vi "Pupil&CR_Detecter.vi"(8 "Image Name":string="ellipse2", 9 "Pupil Threshold":u8=10, 10 "HighLight Spot Threshold":u8=220, 11 "image input":T2) -> (0 "valid fit":T3, 1 "Image Dst Out":T2, 2 "pupil Circles Data":cluster{"Pos. X":sgl, "Pos. Y":sgl}, 3 "CR Circles Data":cluster{"Pos. X":sgl, "Pos. Y":sgl}, 4 "Image Out":T2, 5 "Axis":T1)   [LabVIEW 2011]
uses:
  <vilib>/vision/Image Controls.llb/IMAQ Image.ctl
  <vilib>/vision/NI_Vision_Development_Module.lvlib
panel:
  out "Point 1":cluster{"X":sgl, "Y":sgl}
  out "Point 2":cluster{"X":sgl, "Y":sgl}
  out "CR Valid Fit 2":bool
  out "Pupil Valid Fit":bool
  in  "Size & Tolerance":T4={"X Size"=4, "Y Size"=4, "% Tolerance"=0}
  out "pupil Nb Circles":i32
  in  "CR Max Radius":sgl=10.0 format="%.2f"
  in  "CR Min Radius":sgl=2.0 format="%.2f"
  out "CR Nb Circles":i32
  in  "CR Operator":T5(ring)
  in  "edge Operator":T5(ring)
  in  "edge Range":cluster{"Minimum":sgl, "Maximum":sgl}={"Minimum"=254.0, "Maximum"=255.0} {"Maximum" format="%.2f"; "Minimum" format="%.2f"}
  in  "pupil find edge Method":T6(ring)
  in  "pupil find edge Threshold Value":sgl
  in  "pupil OI Operator":T5(ring)=enum."Square"
  in  "pupil Max Radius":sgl=50.0
  in  "pupil Min Radius":sgl=10.0
  # "step2"
  # "step1"
  # "step1"
  # "step2"
  # "step3"
  # "step4"
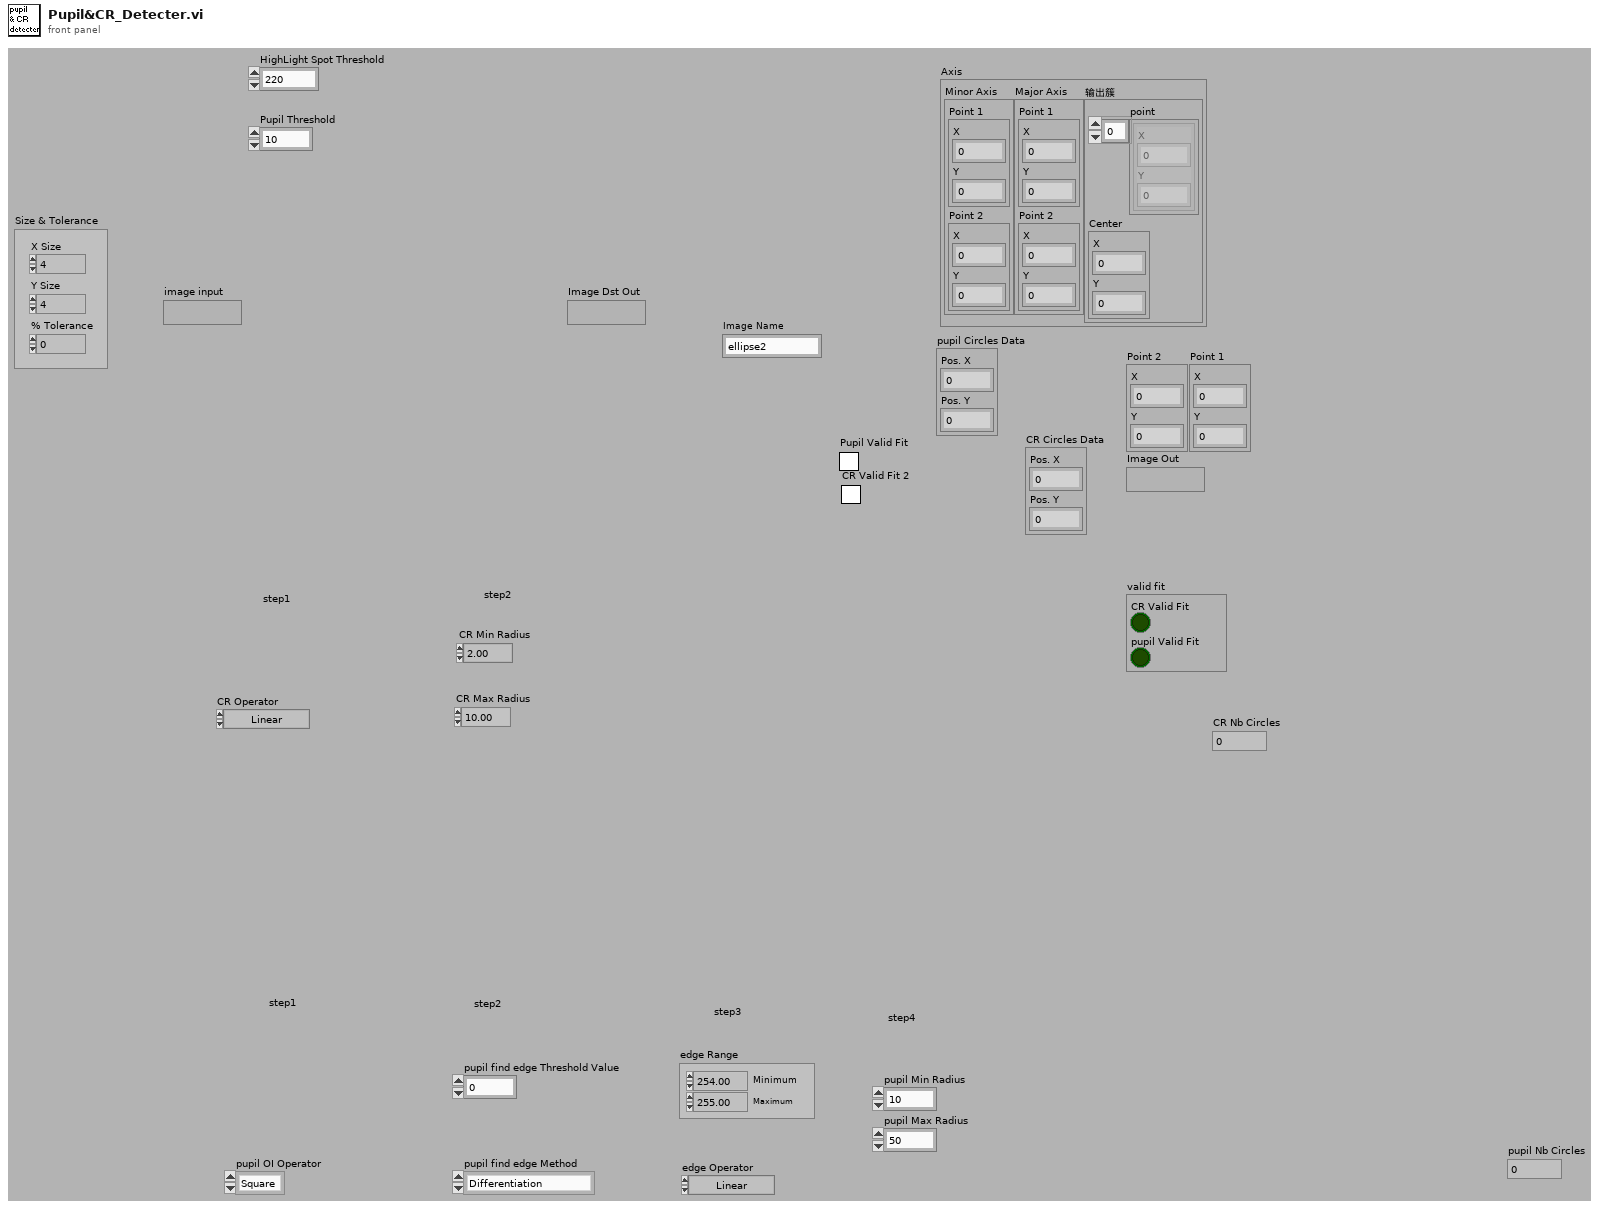
[diagram p1: front panel]
types:
  T1 = cluster{"Minor Axis":cluster{"Point 1":cluster{"X":sgl, "Y":sgl}, "Point 2":cluster{"X":sgl, "Y":sgl}}, "Major Axis":cluster{"Point 1":cluster{"X":sgl, "Y":sgl}, "Point 2":cluster{"X":sgl, "Y":sgl}}, "输出簇":cluster{"point":cluster{"X":i32, "Y":i32}[], "Center":cluster{"X":sgl, "Y":sgl}}}
  T2 = typedef "IMAQ Image.ctl" = refnum<image>
  T3 = cluster{"CR Valid Fit":bool, "pupil Valid Fit":bool}
  T4 = cluster{"X Size":i32, "Y Size":i32, "% Tolerance":i32}
  T5 = enum32{"Linear", "Log", "Exp", "Square", "Square root", "Power X", "Power 1/X"}
  T6 = enum32{"Differentiation", "Gradient", "Prewitt", "Roberts", "Sigma", "Sobel"}
  T7 = typedef "Image Type" = u32
  T8 = cluster{"HighLight Spot Threshold":u8, "Maximum":sgl}
  T9 = cluster{"Pos. X":i32, "Pos. Y":i32, "Radius":i32, "Core Area":i32}[]
  T10 = cluster{"Pos. X":i32, "Pos. Y":i32, "Radius":i32, "Core Area":i32}
  T11 = cluster{"Center":cluster{"X":sgl, "Y":sgl}, "Major Axis":cluster{"Point 1":cluster{"X":sgl, "Y":sgl}, "Point 2":cluster{"X":sgl, "Y":sgl}}, "Minor Axis":cluster{"Point 1":cluster{"X":sgl, "Y":sgl}, "Point 2":cluster{"X":sgl, "Y":sgl}}}
  T12 = cluster{"Point 1":cluster{"X":sgl, "Y":sgl}, "Point 2":cluster{"X":sgl, "Y":sgl}}
  T13 = cluster{"point":cluster{"X":i32, "Y":i32}[], "Center":cluster{"X":sgl, "Y":sgl}}
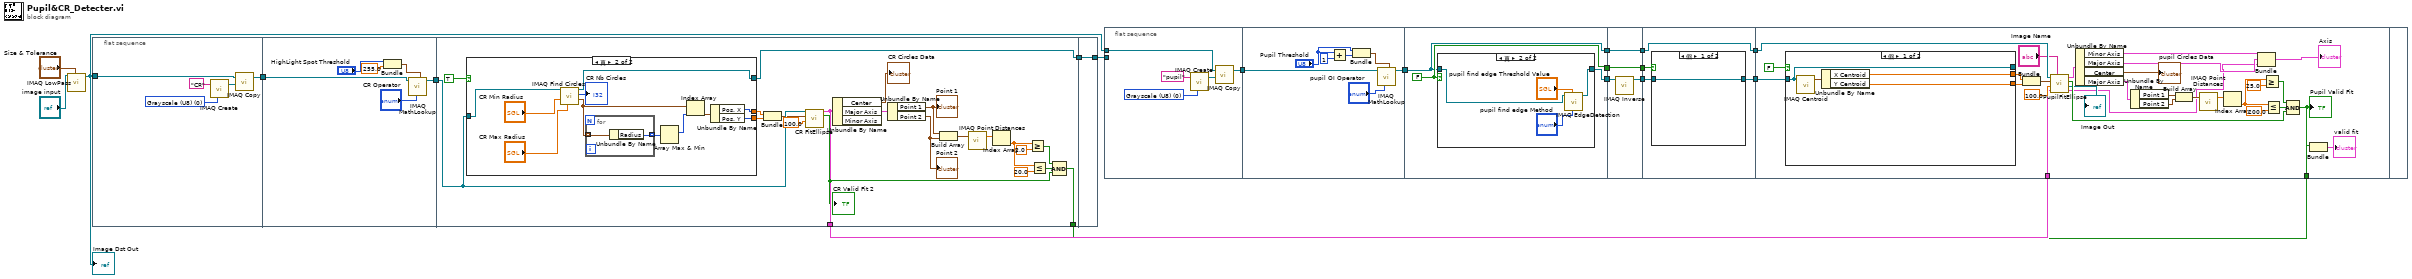
[diagram p0: block diagram]
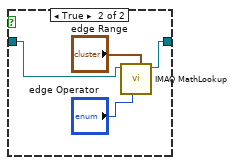
[diagram p3: hidden frame]
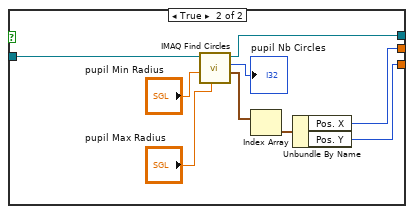
[diagram p4: hidden frame]
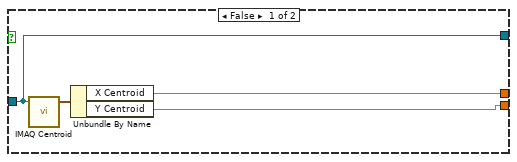
[diagram p5: hidden frame]
diagram:
  n1 = call "IMAQ LowPass"("Image Src"="image input", "Size & Tolerance"="Size & Tolerance") -> ("Image Dst Out"=w8:T2)  [unwired: 3 in, 3 out]
  "Image Dst Out" <- w8
  n2 = flat-sequence {
    tunnel: [w20] -> w12
    tunnel: w8 -> [w21]
    tunnel: [w28] -> w19
    tunnel: w12 -> [w29]
    tunnel: w19 -> [w47]
    tunnel: [w51] -> w18
    tunnel: [w44] -> w3
    tunnel: [w32] -> w1
    tunnel: w18 -> [w69]
    tunnel: [w69] -> w7
    frame #0 {
      w24 = T7 0 items=["Grayscale (U8)", "Grayscale (I16)", "Grayscale (SGL)", "Complex (CSG)", "RGB (U32)", "HSL (U32)", "RGB (U64)", "Grayscale (U16)"] ("Image Type")
      n3 = call "IMAQ Create"("Image Name"="CR", "Image Type"=w24) -> ("New Image"=w23:T2)  [unwired: 2 in, 2 out]
      n4 = call "IMAQ Copy"("Image Dst"=w23, "Image Src"=w21) -> ("Image Dst Out"=w20:T2)  [unwired: 1 in, 4 out]
    }
    frame #1 {
      n5 = Bundle("HighLight Spot Threshold"="HighLight Spot Threshold", "Maximum"=sgl 255.0) -> (w25:T8)  [unwired: 1 out]
      n6 = call "IMAQ MathLookup"("Range"=w25, "Operator"="CR Operator", "Image Src"=w29) -> ("Image Dst Out"=w28:T2)  [unwired: 4 in, 4 out]
    }
    frame #2 {
      n7 = case shown="真" TRUE {
        tunnel: w47 -> [w54 w66]
        tunnel: [w54 w65] -> w51
        tunnel: [w53 w58] -> w50
        tunnel: [w52 w57] -> w49
        frame False {
          n8 = call "IMAQ Centroid"("Image"=w54) -> ("Centroid"=w55:cluster{"X Centroid":sgl, "Y Centroid":sgl})  [unwired: 2 in, 2 out]
          n9 = Unbundle By Name(w55) -> ("X Centroid"=w53:sgl, "Y Centroid"=w52:sgl)
        }
        frame True {
          n10 = call "IMAQ Find Circles"("Max Radius"="CR Max Radius", "Min Radius"="CR Min Radius", "Image Src"=w66) -> ("Circles Data"=w61:T9, "Nb Circles"=→"CR Nb Circles":i32, "Image Dst Out"=w65:T2)  [unwired: 2 in, 4 out]
          n11 = for {
            tunnel: w61 -> [w68] mode=indexing
            tunnel: [w67] -> w60 mode=indexing
            n12 = Unbundle By Name(w68) -> ("Radius"=w67:i32)
          }
          n13 = Array Max & Min(array=w60) -> (max index (indices)=w59:i32)  [unwired: 3 out]
          n14 = Index Array(array=w61, index=w59) -> (element=w56:T10)
          n15 = Unbundle By Name(w56) -> ("Pos. X"=w58:i32, "Pos. Y"=w57:i32)
        }
      }
      n16 = Bundle("X Centroid"=w50, "Y Centroid"=w49) -> (w46:cluster{"X Centroid":sgl, "Y Centroid":sgl})  [unwired: 1 out]
      n17 = call "CR FitEllipse.vi"("r"=100.0, "rough center"=w46, "Image Src"=w47) -> ("Valid Fit"=w33:bool, "Ellipse 2"=w44:T11)  [unwired: 1 in, 6 out]
      "CR Valid Fit 2" <- w33
      n18 = Unbundle By Name(w44) -> ("Center"=→"CR Circles Data":cluster{"X":sgl, "Y":sgl}, "Major Axis"=w43:T12)  [unwired: 1 out]
      n19 = Unbundle By Name(w43) -> ("Point 1"=w42:cluster{"X":sgl, "Y":sgl}, "Point 2"=w41:cluster{"X":sgl, "Y":sgl})
      "Point 2" <- w41
      "Point 1" <- w42
      n20 = Build Array(w42, w41) -> (w40:cluster{"X":sgl, "Y":sgl}[])
      n21 = call "IMAQ Point Distances"("Points"=w40) -> ("Distances"=w39:sgl[])  [unwired: 1 in, 4 out]
      n22 = Index Array(array=w39) -> (element=w37:sgl)  [unwired: 1 in]
      n23 = Greater Or Equal?(x=w37, y=sgl 2.0) -> (x >= y?=w35:bool)
      n24 = Less Or Equal?(x=w37, y=sgl 20.0) -> (x <= y?=w34:bool)
      n25 = Compound Arithmetic op=AND(w35, w34, w33) -> (w32:bool)
    }
    frame #3 {
    }
  }
  n26 = flat-sequence {
    tunnel: [w71] -> w17
    tunnel: w8 -> [w70]
    tunnel: w7 -> [_]
    tunnel: w17 -> [w80]
    tunnel: [w79] -> w16
    tunnel: w16 -> [w82]
    tunnel: [w84] -> w14
    tunnel: [w83] -> w9
    tunnel: [w82] -> w4
    tunnel: w14 -> [w93]
    tunnel: [w92] -> w13
    tunnel: [w91] -> w10
    tunnel: w9 -> [w91]
    tunnel: [w90] -> w5
    tunnel: w4 -> [w90]
    tunnel: [w96] -> w15
    tunnel: w13 -> [w97]
    tunnel: w10 -> [w95]
    tunnel: [w94] -> w6
    tunnel: w5 -> [w94]
    tunnel: w15 -> [w132]
    tunnel: w6 -> [w128]
    tunnel: w3 -> [w124]
    tunnel: w1 -> [w123]
    frame #0 {
      w72 = T7 0 items=["Grayscale (U8)", "Grayscale (I16)", "Grayscale (SGL)", "Complex (CSG)", "RGB (U32)", "HSL (U32)", "RGB (U64)", "Grayscale (U16)"] ("Image Type")
      n27 = call "IMAQ Create"("Image Name"="pupil", "Image Type"=w72) -> ("New Image"=w73:T2)  [unwired: 2 in, 2 out]
      n28 = call "IMAQ Copy"("Image Dst"=w73, "Image Src"=w70) -> ("Image Dst Out"=w71:T2)  [unwired: 1 in, 4 out]
    }
    frame #1 {
      n29 = Add(x="Pupil Threshold", y=u8 1) -> (x+y=w77:u8)
      n30 = Bundle("Pupil Threshold"="Pupil Threshold", w77) -> (w75:cluster{"Pupil Threshold":u8, u8})  [unwired: 1 out]
      n31 = call "IMAQ MathLookup"("Range"=w75, "Operator"="pupil OI Operator", "Image Src"=w80) -> ("Image Dst Out"=w79:T2)  [unwired: 4 in, 4 out]
    }
    frame #2 {
      w83 = FALSE
      n32 = case shown="真" w83 {
        tunnel: w82 -> [w85 w89]
        tunnel: [w85 w86] -> w84
        frame False {
        }
        frame True {
          n33 = call "IMAQ EdgeDetection"("Method"="pupil find edge Method", "Threshold Value"="pupil find edge Threshold Value", "Image Src"=w89) -> ("Image Dst Out"=w86:T2)  [unwired: 3 in, 5 out]
        }
      }
    }
    frame #3 {
      n34 = call "IMAQ Inverse"("Image Src"=w93) -> ("Image Dst Out"=w92:T2)  [unwired: 3 in, 7 out]
    }
    frame #4 {
      n35 = case shown="假" w95 {
        tunnel: w97 -> [w98 w100]
        tunnel: [w98 w99] -> w96
        frame False {
        }
        frame True {
          n36 = call "IMAQ MathLookup"("Range"="edge Range", "Operator"="edge Operator", "Image Src"=w100) -> ("Image Dst Out"=w99:T2)  [unwired: 4 in, 4 out]
        }
      }
    }
    frame #5 {
      n37 = case shown="假" FALSE {
        tunnel: [w136 w145] -> _
        tunnel: w132 -> [w136 w144]
        tunnel: [w134 w138] -> w131
        tunnel: [w133 w137] -> w130
        frame False {
          n38 = call "IMAQ Centroid"("Image"=w136) -> ("Centroid"=w135:cluster{"X Centroid":sgl, "Y Centroid":sgl})  [unwired: 2 in, 2 out]
          n39 = Unbundle By Name(w135) -> ("X Centroid"=w134:sgl, "Y Centroid"=w133:sgl)
        }
        frame True {
          n40 = call "IMAQ Find Circles"("Max Radius"="pupil Max Radius", "Min Radius"="pupil Min Radius", "Image Src"=w144) -> ("Circles Data"=w140:T9, "Nb Circles"=→"pupil Nb Circles":i32, "Image Dst Out"=w145:T2)  [unwired: 2 in, 4 out]
          n41 = Index Array(array=w140) -> (element=w139:T10)  [unwired: 1 in]
          n42 = Unbundle By Name(w139) -> ("Pos. X"=w138:i32, "Pos. Y"=w137:i32)
        }
      }
      n43 = Bundle("X Centroid"=w131, "Y Centroid"=w130) -> (w127:cluster{"X Centroid":sgl, "Y Centroid":sgl})  [unwired: 1 out]
      n44 = call "PupilFitEllipse.vi"("Image Name"="Image Name", "CR Ellipse"=w124, "r"=100.0, "rough center"=w127, "Image Src"=w128) -> ("输出簇"=w103:T13, "Image Out"=→"Image Out":T2, "Valid Fit"=w111:bool, "Ellipse 2"=w125:T11)  [unwired: 3 out]
      n45 = Unbundle By Name(w125) -> ("Minor Axis"=w106:T12, "Major Axis"=w105:T12, "Center"=→"pupil Circles Data":cluster{"X":sgl, "Y":sgl}, "Major Axis"=w112:T12)
      n46 = Unbundle By Name(w112) -> ("Point 1"=w119:cluster{"X":sgl, "Y":sgl}, "Point 2"=w118:cluster{"X":sgl, "Y":sgl})
      n47 = Build Array(w119, w118) -> (w117:cluster{"X":sgl, "Y":sgl}[])
      n48 = call "IMAQ Point Distances"("Points"=w117) -> ("Distances"=w116:sgl[])  [unwired: 1 in, 4 out]
      n49 = Index Array(array=w116) -> (element=w115:sgl)  [unwired: 1 in]
      n50 = Bundle("Minor Axis"=w106, "Major Axis"=w105, "输出簇"=w103) -> (→"Axis":T1)  [unwired: 1 out]
      n51 = Greater Or Equal?(x=w115, y=sgl 25.0) -> (x >= y?=w120:bool)
      n52 = Less Or Equal?(x=w115, y=sgl 200.0) -> (x <= y?=w113:bool)
      n53 = Compound Arithmetic op=AND(w120, w113, w111) -> (w110:bool)
      "Pupil Valid Fit" <- w110
      n54 = Bundle(w123, w110) -> (→"valid fit":cluster{bool, bool})  [unwired: 1 out]
    }
    frame #6 {
    }
  }
